vi "AuMT8852B EDR Sensitivity Extended Results LEG.vi"(5 "Stage":T1(ring), 8 "error in (no error)":errorcluster, 11 "VISA session":refnum<visa-resource-name>) -> (0 "error out":errorcluster, 2 "error code":i32, 3 "VISA session out":refnum<visa-resource-name>, 4 "Results":T2 {"Overall BER" format="%.2e"; "Overall BER" format="%.2e"})   [LabVIEW 2017]
doc: "Anritsu MT8852B Bluetooth Tester\n\n<B>NOTE:</B> USE THIS VI ONLY FOR MT8852B FIRMWARE VERSIONS UP TO AND INCLUDING 4.08.100\n\nReturns the results of the EDR Sensitivity test.\n\nINPUTS\nStage - results of the individual hopping stages of the test.\n\nOUTPUTS\nResults - measurements made during the test."
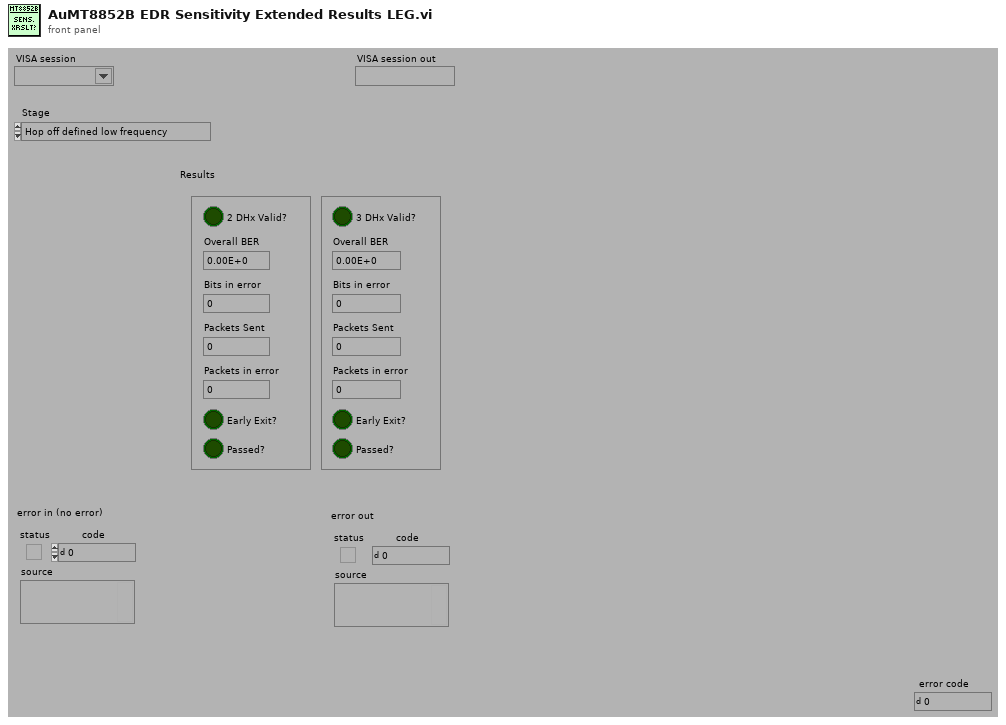
[diagram p1: front panel]
types:
  T1 = enum16{"Hop off defined low frequency", "Hop off defined medium frequency", "Hop off defined high frequency", "Hop on any channels"}
  T2 = cluster{"2 DHx Valid?":bool, "Overall BER":dbl, "Bits in error":u32, "Packets Sent":u32, "Passed?":bool, "Packets in error":u32, "Early Exit?":bool, "3 DHx Valid?":bool, "Overall BER":dbl, "Bits in error":u32, "Packets Sent":u32, "Passed?":bool, "Packets in error":u32, "Early Exit?":bool}
  T3 = enum16{"Simulate", "Range check", "Cache", "Query instrument status"}
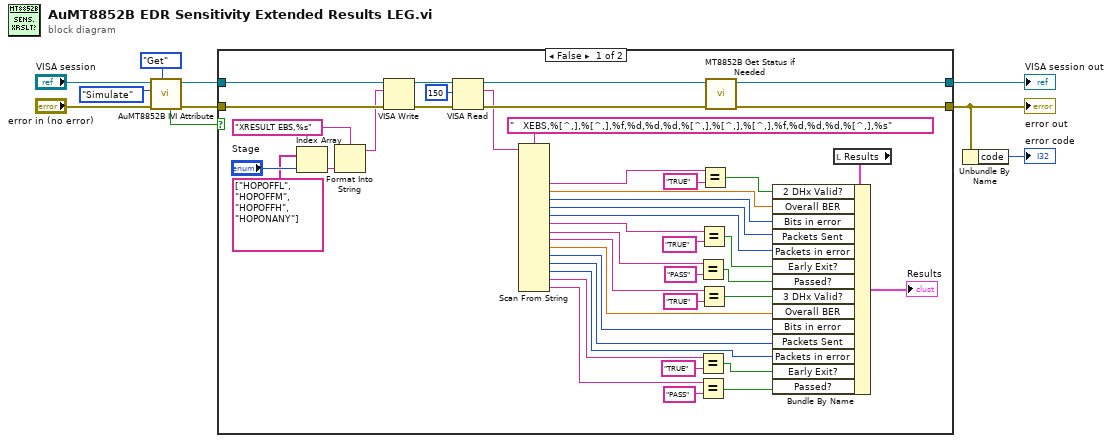
[diagram p0: block diagram]
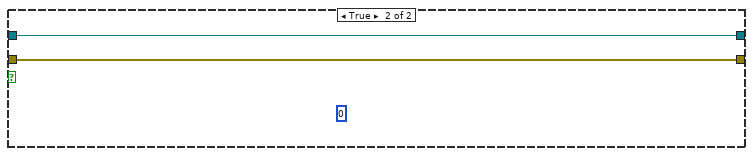
[diagram p2: hidden frame]
diagram:
  n1 = call <instrlib>:"AuMT8852B IVI Attribute.vi"("Set/Get (Set)"=enum16{"Set", "Get"}."Get", "error in (no error)"="error in (no error)", "Flag (Simulate)"=T3."Simulate", "VISA session"="VISA session") -> ("error out"=w7:errorcluster, "VISA session out"=w9:refnum<visa-resource-name>, "Value out"=w3:bool)  [unwired: 5 in]
  n2 = case shown="False" w3 {
    tunnel: [w48 w56] -> w10
    tunnel: [w47 w55] -> w1
    tunnel: w9 -> [w54 w56]
    tunnel: w7 -> [w53 w55]
    frame False {
      n3 = Index Array(array=string[] ["HOPOFFL", "HOPOFFM", "HOPOFFH", "HOPONANY"], index="Stage") -> (element=w39:string)
      n4 = Format Into String(format string="XRESULT EBS,%s" ("write buffer (\"\")"), w39) -> (resulting string=w36:string)  [unwired: 2 in, 1 out]
      n5 = VISA Write(VISA resource name=w54, write buffer=w36, error in (no error)=w53) -> (VISA resource name out=w52:refnum<visa-resource-name>, error out=w51:errorcluster)  [unwired: 1 out]
      n6 = VISA Read(VISA resource name=w52, byte count=u32 150 ("byte count (0)"), error in (no error)=w51) -> (VISA resource name out=w46:refnum<visa-resource-name>, read buffer=w34:string, error out=w45:errorcluster)  [unwired: 1 out]
      n7 = Scan From String(format string="   XEBS,%[^,],%[^,],%f,%d,%d,%d,%[^,],%[^,],%[^,],%f,%d,%d,%d,%[^,],%s" ("Format String"), input string=w34) -> (output 2=w33:string, output 3=w18:dbl, output 4=w17:i32, output 5=w20:i32, output 6=w19:i32, output 7=w11:string, output 8=w32:string, output 9=w12:string, output 10=w21:dbl, output 11=w22:i32, output 12=w23:i32, output 13=w24:i32, output 14=w25:string, output 15=w31:string)  [unwired: 18 in, 3 out]
      n8 = Equal?(x=w32, y="PASS") -> (x = y?=w15:bool)
      n9 = Equal?(x=w25, y="TRUE") -> (x = y?=w26:bool)
      n10 = Equal?(x=w31, y="PASS") -> (x = y?=w28:bool)
      n11 = Equal?(x=w11, y="TRUE") -> (x = y?=w16:bool)
      n12 = Equal?(x=w12, y="TRUE") -> (x = y?=w13:bool)
      n13 = Equal?(x=w33, y="TRUE") -> (x = y?=w44:bool)
      n14 = call <instrlib>:"MT8852B Get Status if Needed.vi"("error in (no error)"=w45, "VISA session"=w46) -> ("error out"=w47:errorcluster, "VISA session out"=w48:refnum<visa-resource-name>)  [unwired: 8 in]
      n15 = local read "Results"() -> (w30:T2)
      n16 = Bundle By Name(cluster=w30, "2 DHx Valid?"=w44, "Overall BER"=w18, "Bits in error"=w17, "Packets Sent"=w20, "Packets in error"=w19, "Early Exit?"=w16, "Passed?"=w15, "3 DHx Valid?"=w13, "Overall BER"=w21, "Bits in error"=w22, "Packets Sent"=w23, "Packets in error"=w24, "Early Exit?"=w26, "Passed?"=w28) -> (→"Results":T2)
    }
    frame True {
      (unwired) u8 0
    }
  }
  "error out" <- w1
  "VISA session out" <- w10
  n17 = Unbundle By Name(w1) -> ("code"=→"error code":i32)
